vi "dBScale.vi"(4 "Bit Depth":i32=8, 5 "Data In":dbl[][](array[numeric])) -> (2 "Data Out":dbl[][](array[numeric]))   [LabVIEW 2022 SP3]
uses:
  <vilib>/Analysis/NI_AALPro.lvlib
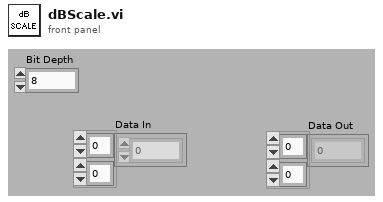
[diagram p1: front panel]
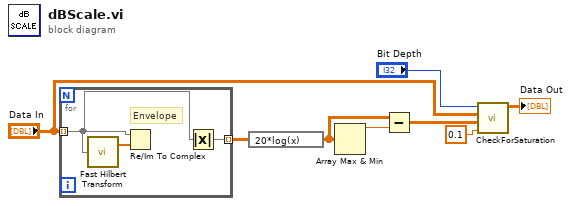
[diagram p0: block diagram]
diagram:
  n1 = for {
    tunnel: "Data In" -> [w9] mode=indexing
    tunnel: [w11] -> w7 mode=indexing
    # "Envelope"
    n2 = call <vilib>:"Fast Hilbert Transform.vi"("X"=w9) -> ("Hilbert{X}"=w10:dbl[])  [unwired: 1 out]
    n3 = Re/Im To Complex(1:w10, 2:w9) -> ()  [unwired: 1 out]
    n4 = Absolute Value(x=w9) -> (abs(x)=w11:dbl[])
  }
  n5 = expression code="20*log(x)"(w7) -> (w8:dbl[][])
  n6 = Array Max & Min(array=w8) -> (max value=w6:dbl)  [unwired: 3 out]
  n7 = Subtract(x=w8, y=w6) -> (x-y=w5:dbl[][])
  n8 = call "CheckForSaturation.vi"("Replace Sat with X?"=0.1, "Processed Data"=w5, "Original Data In"="Data In", "Bit Depth"="Bit Depth") -> ("Data with Saturation"=→"Data Out":dbl[][])  [unwired: 7 in]
